vi "Client.vi"() -> ()   [LabVIEW 2020]
panel:
  out "data out":string
  in  "Boolean":bool
  in  "stop":bool
  out "error out":errorcluster
  out "String":string
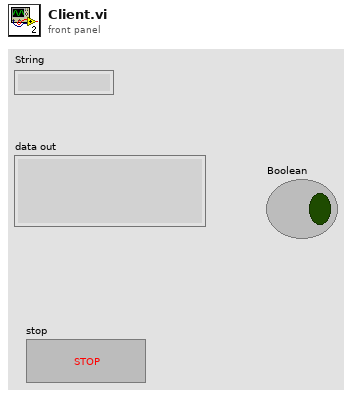
[diagram p1: front panel]
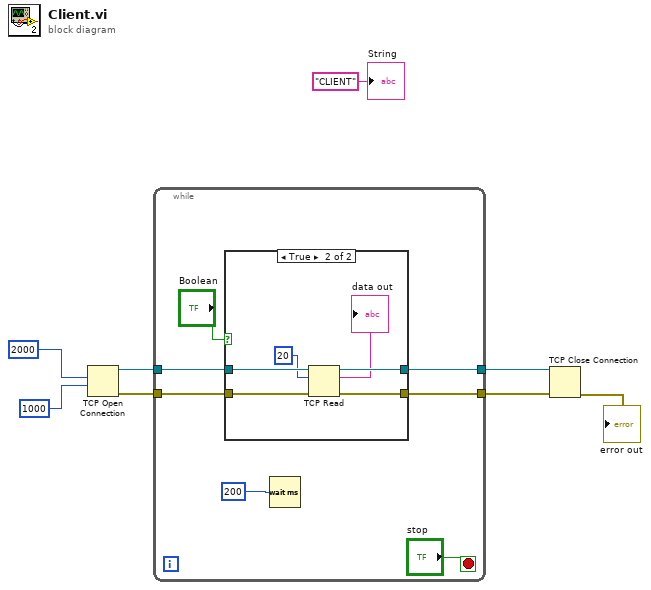
[diagram p0: block diagram]
diagram:
  n1 = TCP Open Connection(remote port or service name=u16 2000, timeout ms (60000)=1000) -> (connection ID=w4:refnum<k5>, error out=w5:errorcluster)  [unwired: 3 in]
  n2 = while {
    tunnel: w4 -> [w14]
    tunnel: [w13] -> w3
    tunnel: w5 -> [w15]
    tunnel: [w12] -> w2
    stop <- "stop" stop-if-true
    n3 = case shown="True" "Boolean" {
      tunnel: w15 -> [_ w21]
      tunnel: w14 -> [_ w20]
      tunnel: [_ w19] -> w13
      tunnel: [_ w18] -> w12
      frame False {
      }
      frame True {
        n4 = TCP Read(connection ID=w20, bytes to read=20, error in (no error)=w21) -> (connection ID out=w19:refnum<k5>, data out=→"data out":string, error out=w18:errorcluster)  [unwired: 2 in]
      }
    }
    n5 = Wait (ms)(milliseconds to wait=u32 200) -> ()  [unwired: 1 out]
  }
  n6 = TCP Close Connection(connection ID=w3, error in (no error)=w2) -> (error out=→"error out":errorcluster)  [unwired: 1 in, 1 out]
  "String" <- "CLIENT" ("String")
